vi "loadSubVI.vi"(8 "error in":errorcluster, 9 "Node Path":string, 10 "RootNode*":refnum<data-value>, 11 "SubPanel in":refnum<class "xceSubPanel.lvclass">) -> (0 "error out":errorcluster, 3 "SubPanel":refnum<class "xceSubPanel.lvclass">)   [LabVIEW 2013, in "xceSubPanel.lvclass"]
doc: "Starts a xceCnfgItems UI VI, and then inserts it into the subpanel."
uses:
  xceSubPanel.lvclass
  xceRootNode/xceRootNode.lvclass
  xceDataNode/xceDataNode.lvclass
  xceSubPanel.lvclass/xceSubPanel.ctl
  xceNode/xceNode.lvclass
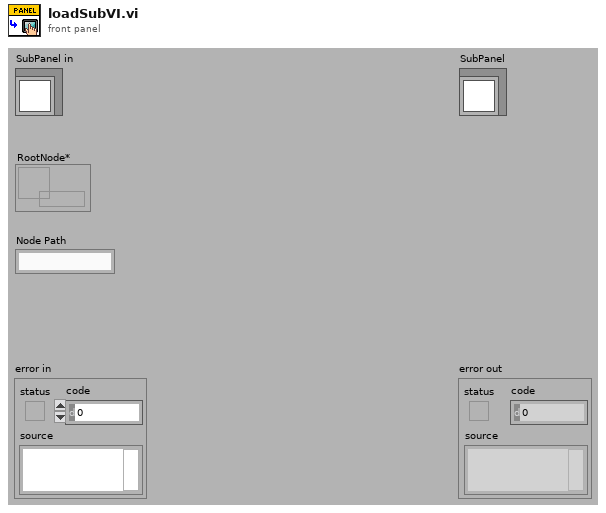
[diagram p1: front panel]
types:
  T1 = typedef "AMC.lvlib/Message Queue.ctl" = refnum<queue>
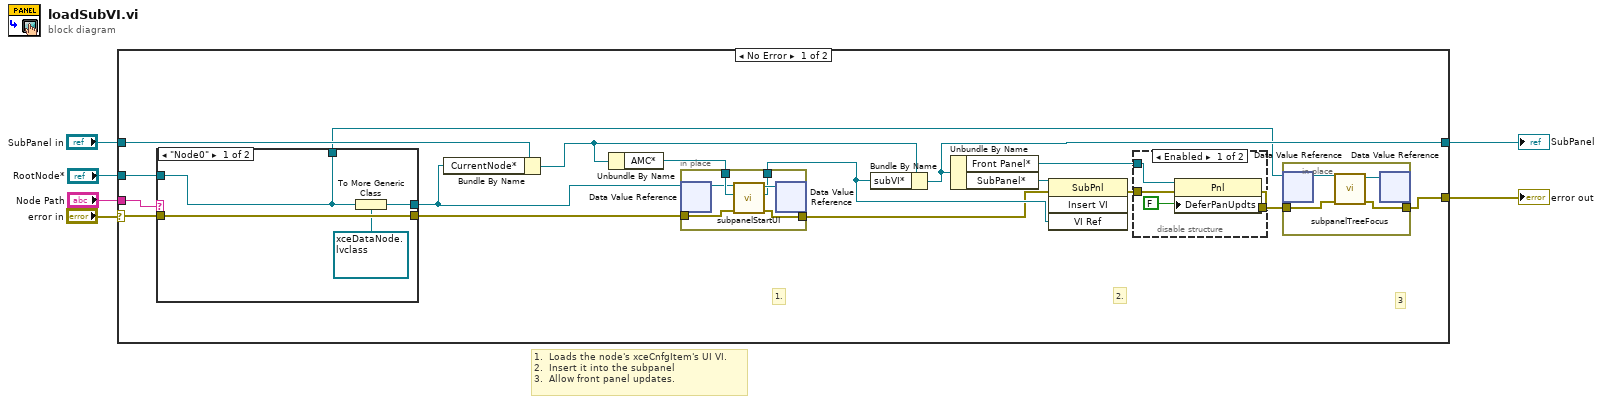
[diagram p0: block diagram]
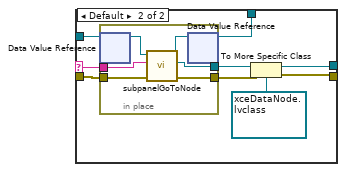
[diagram p3: hidden frame]
diagram:
  # "1.  Loads the node's xceCnfgItem's UI VI.\n2.  Insert it into the subpanel\n3.  Allow front panel updates."
  n1 = case shown="No Error" "error in" {
    selector: "error in" -> [w21 w59]
    tunnel: [w7 w59] -> w5
    tunnel: [w14 w58] -> w3
    tunnel: "SubPanel in" -> [w23 w58]
    tunnel: "Node Path" -> [w20 _]
    tunnel: "RootNode*" -> [w19 _]
    frame No Error {
      # "3"
      # "2."
      # "1."
      n2 = case shown="\"Node0\"" w20 {
        selector: w20 -> [_ w50]
        tunnel: w21 -> [w42 w51]
        tunnel: [w39 w45] -> w18
        tunnel: [w42 w44] -> w13
        tunnel: w19 -> [w41 w49]
        tunnel: [w41 w43] -> w11
        frame "Node0" {
          n3 = To More Generic Class(target class=refnum<data-value> refnum ("RootNode* in"), reference=w41) -> (generic class reference=w39:refnum<data-value>)
        }
        frame Default {
          n4 = in-place {
            in-place-border: w51 -> [w56]
            in-place-border: w50 -> [w53]
            in-place-border: [w52] -> w46
            in-place-border: [w55] -> w47
            n5 = in-place-dvr #1(w49) -> (w57:refnum<class "xceRootNode.lvclass">)  [unwired: 1 out]
            n6 = call "subpanelGoToNode.vi"("error in (no error)"=w56, "Node Path"=w53, "xceNode in"=w57) -> ("error out"=w55:errorcluster, "goToNode* out"=w52:refnum<data-value>, "xceNode out"=w54:refnum<class "xceRootNode.lvclass">)  [unwired: 6 in]
            n7 = in-place-dvr #1(w54) -> (w43:refnum<data-value>)  [unwired: 1 out]
          }
          n8 = To More Specific Class(target class=refnum<data-value> refnum ("RootNode* in"), reference=w46, error in=w47) -> (specific class reference=w45:refnum<data-value>, error out=w44:errorcluster)
        }
      }
      n9 = Bundle By Name(cluster=w23, "CurrentNode*"=w18) -> (w15:refnum<class "xceSubPanel.lvclass">)
      n10 = Unbundle By Name(w15) -> ("AMC*"=w17:T1)
      n11 = in-place {
        in-place-border: w13 -> [w37]
        in-place-border: [w36] -> w12
        in-place-border: w17 -> [w35]
        in-place-border: [w34] -> w16
        n12 = in-place-dvr #2(w18) -> (w33:refnum<class "xceDataNode.lvclass">)  [unwired: 1 out]
        n13 = call "subpanelStartUI.vi"("error in (no error)"=w37, "AMC*"=w35, "xceDataNode in"=w33) -> ("error out"=w36:errorcluster, "UI VI*"=w34:refnum<vi>, "xceDataNode out"=w38:refnum<class "xceDataNode.lvclass">)  [unwired: 6 in]
        n14 = in-place-dvr #2(w38) -> ()  [unwired: 2 out]
      }
      n15 = Bundle By Name(cluster=w15, "subVI*"=w16) -> (w14:refnum<class "xceSubPanel.lvclass">)
      n16 = Unbundle By Name(w14) -> ("Front Panel*"=w10:refnum<vi>, "SubPanel*"=w22:refnum<vi>)
      n17 = invoke class="SubPnl" method="Insert VI"(reference=w22, error in=w12, "VI Ref"=w16) -> (error out=w9:errorcluster)  [unwired: 1 in, 3 out]
      n18 = disable-structure shown="Enabled" {
        disable-tunnel: w10 -> [w26 _]
        disable-tunnel: w9 -> [w25 w28]
        disable-tunnel: [w24 w28] -> w8
        frame Enabled {
          n19 = property class="Pnl"(reference=w26, error in=w25, "DeferPanUpdts"=FALSE ("Defer Panel Updates")) -> (error out=w24:errorcluster)  [unwired: 1 out]
        }
        frame Disabled {
        }
      }
      n20 = in-place {
        in-place-border: w8 -> [w30]
        in-place-border: [w29] -> w7
        n21 = in-place-dvr #3(w11) -> (w32:refnum<class "xceRootNode.lvclass">)  [unwired: 1 out]
        n22 = call "subpanelTreeFocus.vi"("error in (no error)"=w30, "xceRootNode in"=w32) -> ("error out"=w29:errorcluster, "xceRootNode out"=w31:refnum<class "xceRootNode.lvclass">)  [unwired: 8 in]
        n23 = in-place-dvr #3(w31) -> ()  [unwired: 2 out]
      }
    }
    frame Error {
    }
  }
  "error out" <- w5
  "SubPanel" <- w3
